vi "XNET TCP Socket Create Listener.vi"(6 "local interface":string, 7 "stack":refnum<k21>, 8 "error in":errorcluster, 9 "timeout ms (25000)":i32=25000, 10 "local port":u16) -> (0 "error out":errorcluster, 2 "actual local port":u16, 3 "listener socket":refnum<k20>)   [LabVIEW 2018]
doc: "Use this node with XNET TCP Socket Wait on Listener to create and listen for connections on the server."
uses:
  nixlvapi.dll
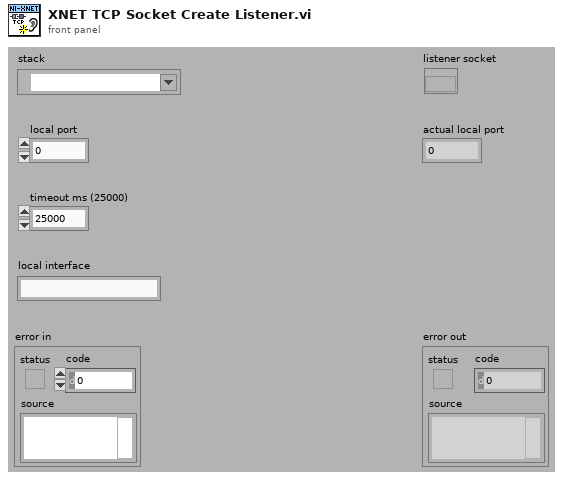
[diagram p1: front panel]
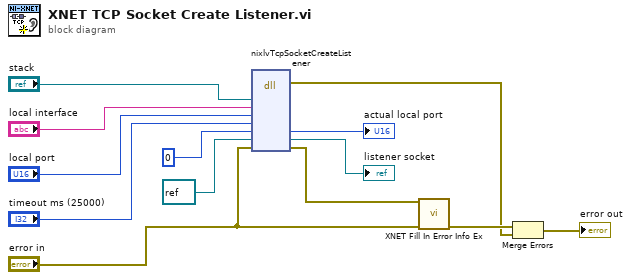
[diagram p0: block diagram]
diagram:
  n1 = dll-call lib="nixlvapi.*" fn="nixlvTcpSocketCreateListener" label="Call Library"("stackRef"="stack", "localInterface"="local interface", "localPort"="local port", "timeoutMs"="timeout ms (25000)", "actualLocalPort"=u16 0, "socketRefObjPtr"=refnum<k20> refnum ("listener socket"), "errorInOut"="error in") -> (error out=w11:errorcluster, "actualLocalPort"=→"actual local port":u16, "socketRefObjPtr"=→"listener socket":refnum<k20>, "errorInOut"=w13:errorcluster)  [unwired: 3 in, 6 out]
  n2 = call "XNET Fill In Error Info Ex.vi"("error xnet"=w13, "error in"="error in") -> ("error out"=w12:errorcluster)  [unwired: 13 in]
  n3 = Merge Errors(w12, w11) -> (→"error out":errorcluster)
